vi "setNormLUT.vi"(2 "Frequency":dbl=1000.0, 3 "Number of entries in LUT":dbl=512.0, 4 "Count":dbl) -> (0 "Time to wait (s)":dbl, 1 "Normalized bin":u32)   [LabVIEW 2012]
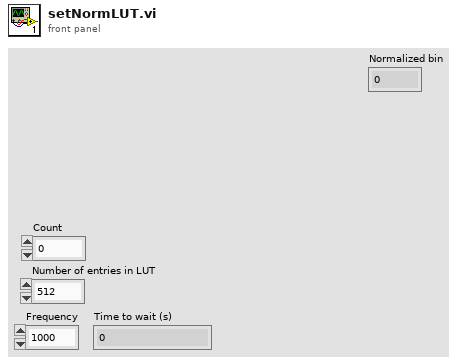
[diagram p1: front panel]
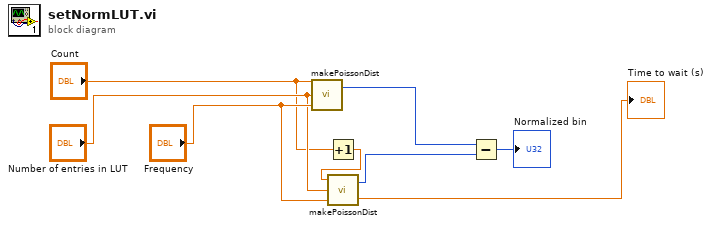
[diagram p0: block diagram]
diagram:
  n1 = call "makePoissonDist.vi"("Frequency"="Frequency", "Number of entries in LUT"="Number of entries in LUT", "Input"="Count") -> ("Output"=w4:u32)  [unwired: 1 out]
  n2 = Increment(x="Count") -> (x+1=w5:dbl)
  n3 = call "makePoissonDist.vi"("Frequency"="Frequency", "Number of entries in LUT"="Number of entries in LUT", "Input"=w5) -> ("Time to wait (s)"=→"Time to wait (s)":dbl, "Output"=w3:u32)
  n4 = Subtract(x=w4, y=w3) -> (x-y=→"Normalized bin":u32)
